vi "1-Tap 8-Bit Camera with Centroid (Host).vi"() -> ()   [LabVIEW 2012]
doc: "This is the host VI for the 1-Tap 8-Bit Camera with Centroid example. This example demonstrates how to perform image processing operations on the FPGA in real time and display the results on the host. This example performs an image thresholding operation followed by a centroid computation. The threshold parameters can be modified using the controls on the front panel. The thresholded images and centroid coordinates are displayed in real time.\n\nAdditionally, the example demonstrates the serial server, which allows third-party camera configuration utilities to communicate with the camera using the Camera Link serial interface while this VI is running."
uses:
  <vilib>/userdefined/High Color/nirio_resource_hc.ctl
  <vilib>/FPGAPlugInAG/PCIe-1473R/niLvFpga_Open_PCIe-1473R.vi
  <vilib>/rvi/interface/common/dynamic/niFpgaDynamicAddResources.vi
  <vilib>/FPGAPlugInAG/Dynamic/niLvFpga_Reset_Dynamic.vi
  <vilib>/Utility/error.llb/Error Cluster From Error Code.vi
  <vilib>/rvi/errors/niLvFpgaAdjustHostInterfaceError.vi
  <vilib>/FPGAPlugInAG/Dynamic/niLvFpga_Run_Dynamic.vi
  <vilib>/FPGAPlugInAG/Dynamic/niLvFpga_Close_Dynamic.vi
  <vilib>/rvi/interface/nirviOpenFPGA/nirviOpenFPGA.xnode
  FPGA Bitfiles/1-Tap8-BitCamera_FPGATarget_1-Tap8-BitCamera_B0CF732A.lvbitx
  1-Tap 8-Bit Camera with Centroid (FPGA).vi
  <vilib>/rvi/interface/nirviMethod/nirviMethod.xnode
  <vilib>/rvi/interface/nirviReadWriteControl/nirviReadWriteControl.xnode
  <vilib>/rvi/interface/nirviCloseFPGA/nirviCloseFPGA.xnode
  NiFpgaLv.dll
  <vilib>/rvi/interface/Simulation/niFpgaSimulationCallBeginRW.vi
  <vilib>/FPGAPlugInAG/Dynamic/niLvFpga_ConfigureFifo_Dynamic.vi
  <vilib>/rvi/errors/niLvFpgaMergeErrorWithErrorCode.vi
  <vilib>/FPGAPlugInAG/Dynamic/niLvFpga_StartFifo_Dynamic.vi
  <vilib>/FPGAPlugInAG/Dynamic/niLvFpga_ReadFifo_Dynamic.vi
panel:
  in  "Invert Image":bool
  out "Y Centroid":fxp<+,32,16> format="%.21g"
  out "X Centroid":fxp<+,32,16> format="%.21g"
  in  "Replace?":bool
  in  "Replace Value":u8=255
  in  "Lower Limit":u8=128
  in  "Upper Limit":u8=255
  out "Acq In Progress":bool
  in  "Line Scan":bool
  in  "Frames To Acquire":u32=1 caption="Frames To Acquire\n(0 = infinite)"
  in  "Cancel":bool
  out "Acq'd Frame Width":u32
  in  "Stopped":bool
  in  "RIO Device":T1="RIO0"
  out "DMA Write Timeout":bool
  in  "Start Serial Server":bool=TRUE
  out "Frames Acq'd":u32
  out "Acq'd Frame Height":u32
  out "Image":T2(plugin-control)
  in  "Acquire":bool
  in  "Stop":bool
  in  "Image Height":u32=480 max=65535
  in  "Image Width":u32=640 max=65535
  out "Initialized":bool
  # "Note: For the centroid, the image must be a light object\non dark background, or you can invert the image."
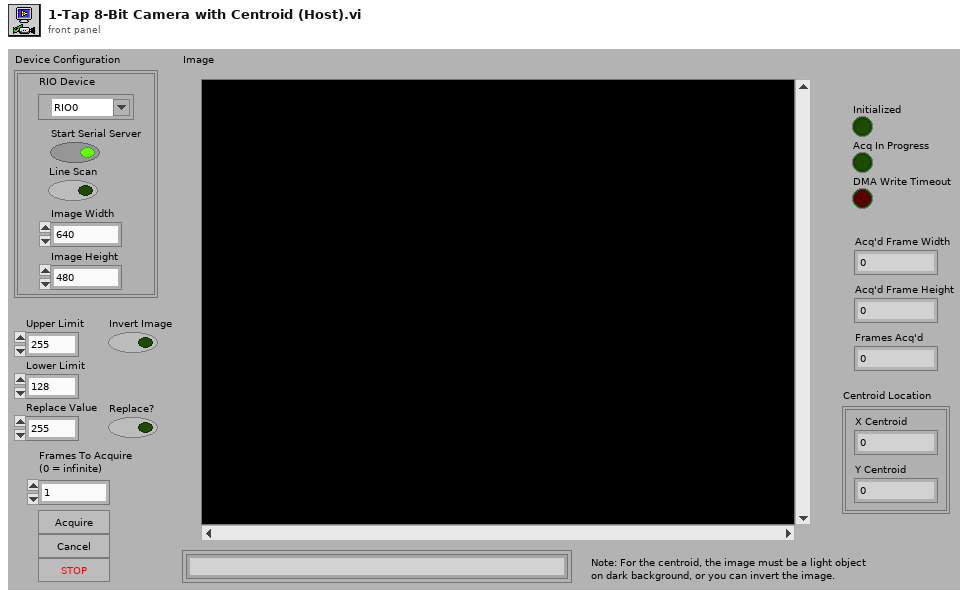
[diagram p1: front panel]
types:
  T1 = typedef "nirio_resource_hc.ctl" = tag
  T2 = typedef "IMAQ Image.ctl" = refnum<image>
  T3 = enum8{"Standard", "Basler 10-tap", "Vosskühler 10-tap"}
  T4 = typedef "Image Type" = u32
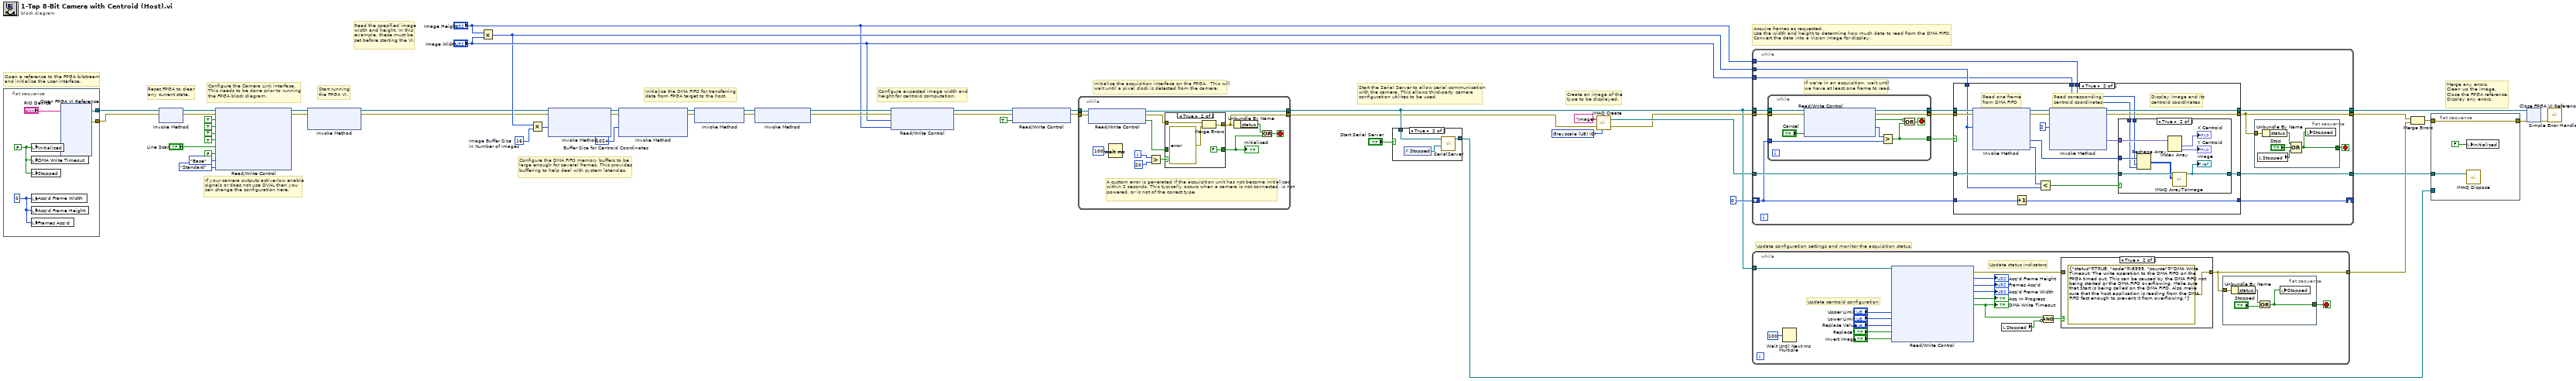
[diagram p0: block diagram]
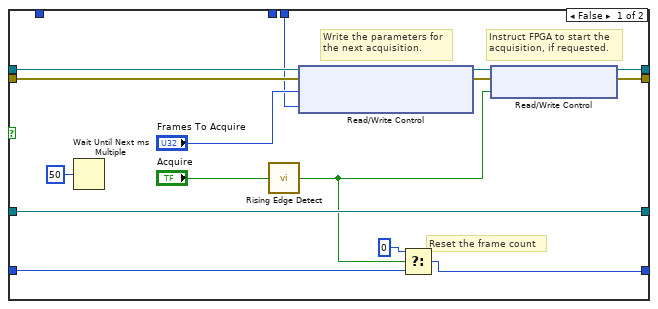
[diagram p4: hidden frame]
diagram:
  w10 = 1024  # Buffer Size for Centroid Coordinates
  w47 = T4 0 items=["Grayscale (U8)", "Grayscale (I16)", "Grayscale (SGL)", "Complex (CSG)", "RGB (U32)", "HSL (U32)", "RGB (U64)", "Grayscale (U16)"] ("Image Type")
  w28 = u32 16  # Image Buffer Size in Number of Images
  # "Configure expected image width and\nheight for centroid computation."
  # "If your camera outputs active-low enable\nsignals or does not use DVAL then you\ncan change the configuration here."
  # "Configure the DMA FIFO memory buffers to be\nlarge enough for several frames. This provides\nbuffering to help deal with system latencies."
  # "Start running\nthe FPGA VI."
  # "Reset FPGA to clear\nany current state."
  # "Read the specified image\nwidth and height. In this\nexample, these must be\nset before starting the VI."
  # "Merge any errors.\nClean up the image.\nClose the FPGA reference.\nDisplay any errors."
  # "Acquire frames as requested.\nUse the width and height to determine how much data to read from the DMA FIFO.\nConvert the data into a Vision Image for display."
  # "Update configuration settings and monitor the acquisition status."
  # "Start the Serial Server to allow serial communication\nwith the camera. This allows third-party camera\nconfiguration utilites to be used."
  # "Create an image of the\ntype to be displayed."
  # "Initialize the acquisition interface on the FPGA.  This will\nwait until a pixel clock is detected from the camera."
  # "Initialize the DMA FIFO for transferring\ndata from FPGA target to the host."
  # "Configure the Camera Link interface.\nThis needs to be done prior to running\nthe FPGA block diagram."
  # "Open a reference to the FPGA bitstream\nand initialize the user interface."
  n1 = flat-sequence {
    tunnel: [w53] -> w43
    tunnel: [w52] -> w51
    frame #0 {
      w56 = u32 0 ("Num Lines Acq'd")
      w55 = FALSE ("stop")
      n2 = local write "Initialized"(w55) -> ()
      n3 = local write "DMA Write Timeout"(w55) -> ()
      n4 = local write "Stopped"(w55) -> ()
      n5 = local write "Acq'd Frame Width"(w56) -> ()
      n6 = local write "Acq'd Frame Height"(w56) -> ()
      n7 = local write "Frames Acq'd"(w56) -> ()
      n8 = xnode "Open FPGA VI Reference"("resource name"="RIO Device") -> ("FPGA VI Reference Out"=w53:refnum<k20>, "error out"=w52:errorcluster)  [unwired: 1 in]
    }
  }
  n9 = xnode "Invoke Method"("FPGA VI Reference In"=w43, "error in"=w51) -> ("FPGA VI Reference Out"=w35:refnum<k20>, "error out"=w38:errorcluster)
  n10 = xnode "Read/Write Control"("FPGA VI Reference In"=w35, "error in"=w38, "CL Config.FVAL Active High"=TRUE ("IO Module Config.CL FVAL Active High"), "CL Config.LVAL Active High"=TRUE ("IO Module Config.CL LVAL Active High"), "CL Config.DVAL Active High"=TRUE ("IO Module Config.CL DVAL Active High"), "CL Config.Spare Active High"=TRUE ("IO Module Config.CL Spare Active High"), "CL Config.Line Scan"="Line Scan", "Acq Control.Ignore DVAL"=FALSE ("CL Config.Line Scan"), "CL Config.Configuration"=enum8{"Base", "Medium", "Full"}."Base", "CL Config.Signal Mapping"=T3."Standard") -> ("FPGA VI Reference Out"=w39:refnum<k20>, "error out"=w37:errorcluster)
  n11 = xnode "Invoke Method"("FPGA VI Reference In"=w39, "error in"=w37) -> ("FPGA VI Reference Out"=w2:refnum<k20>, "error out"=w1:errorcluster)  [unwired: 1 in]
  n12 = Multiply(x="Image Height", y="Image Width") -> (x*y=w11:u32)
  n13 = Multiply(x=w11, y=w28) -> (x*y=w30:u32)
  n14 = xnode "Invoke Method"("FPGA VI Reference In"=w2, "error in"=w1, "Requested Depth"=w30) -> ("FPGA VI Reference Out"=w23:refnum<k20>, "error out"=w20:errorcluster)  [unwired: 1 out]
  n15 = xnode "Invoke Method"("FPGA VI Reference In"=w23, "error in"=w20, "Requested Depth"=w10) -> ("FPGA VI Reference Out"=w22:refnum<k20>, "error out"=w19:errorcluster)  [unwired: 1 out]
  n16 = xnode "Invoke Method"("FPGA VI Reference In"=w22, "error in"=w19) -> ("FPGA VI Reference Out"=w21:refnum<k20>, "error out"=w18:errorcluster)
  n17 = xnode "Invoke Method"("FPGA VI Reference In"=w21, "error in"=w18) -> ("FPGA VI Reference Out"=w17:refnum<k20>, "error out"=w16:errorcluster)
  n18 = xnode "Read/Write Control"("FPGA VI Reference In"=w17, "error in"=w16, "Centroid.Image Width"="Image Width", "Centroid.Image Height"="Image Height") -> ("FPGA VI Reference Out"=w13:refnum<k20>, "error out"=w12:errorcluster)
  n19 = xnode "Read/Write Control"("FPGA VI Reference In"=w13, "error in"=w12, "Acq Control.Initialize"=TRUE ("Arm Acquisition")) -> ("FPGA VI Reference Out"=w50:refnum<k20>, "error out"=w49:errorcluster)
  n20 = while {
    tunnel: w50 -> [w64]
    tunnel: w49 -> [w63]
    tunnel: [w62] -> w27
    tunnel: [w66] -> w26
    i -> [w58]
    stop <- w69 stop-if-true
    # "A custom error is generated if the acquisition unit has not become initialized within 2 seconds. This typically occurs when a camera is not connected, is not powered, or is not of the correct type."
    n21 = xnode "Read/Write Control"("FPGA VI Reference In"=w64, "error in"=w63) -> ("FPGA VI Reference Out"=w62:refnum<k20>, "error out"=w61:errorcluster, "Acq Status.Initialized"=w60:bool)
    n22 = Wait (ms)(milliseconds to wait=u32 100) -> ()  [unwired: 1 out]
    n23 = Greater?(x=w58, y=20) -> (0:w59:bool)
    n24 = case shown="True" w59 {
      tunnel: [w71 FALSE] -> w65
      tunnel: w60 -> [w71 _]
      tunnel: w61 -> [w70 w73]
      tunnel: [w70 w75] -> w66
      frame False {
      }
      frame True {
        n25 = Merge Errors(w73, errorcluster {"status"=TRUE, "code"=-8999, "source"="Acquisition Initialization: This error typically occurs when a camera is not properly connected, is not powered, or is not of the correct type."} ("error in")) -> (w75:errorcluster)
      }
    }
    "Initialized" <- w65
    n26 = Unbundle By Name(w66) -> ("status"=w68:bool)
    n27 = Or(x=w68, y=w65) -> (x .or. y?=w69:bool)
  }
  n28 = case shown="True" "Start Serial Server" {
    tunnel: [_ w76] -> w44
    tunnel: w27 -> [_ w77]
    frame False {
    }
    frame True {
      n29 = control-ref of="Stopped"() -> (w78:refnum<vi>)
      n30 = call "SerialServer.vi"("Stop Refnum"=w78, "FPGA VI Reference In"=w77) -> ("FPGA VI Reference Out"=w76:refnum<k20>)  [unwired: 5 in]
    }
  }
  n31 = call "IMAQ Create"("Image Name"="Image", "Image Type"=w47, "error in (no error)"=w26) -> ("New Image"=w6:T2, "error out"=w5:errorcluster)  [unwired: 2 in]
  n32 = while {
    tunnel: w27 -> [w85]
    tunnel: w5 -> [w84]
    tunnel: w11 -> [w93]
    tunnel: "Image Height" -> [w92]
    tunnel: "Image Width" -> [w91]
    tunnel: w6 -> [w90]
    tunnel: [w88] -> w41
    tunnel: [w89] -> w9
    tunnel: [w86] -> w45
    shift-right: [w80] -> _
    shift-left: u32 0 -> [w79]
    stop <- w87 stop-if-true
    # "If we're in an acquisition, wait until\nwe have at least one frame to read."
    n33 = while {
      tunnel: w85 -> [w100]
      tunnel: w84 -> [w99]
      tunnel: [w97] -> w83
      tunnel: [w98] -> w82
      tunnel: w79 -> [w103]
      tunnel: [w101] -> w81
      stop <- w102 stop-if-true
      n34 = xnode "Read/Write Control"("FPGA VI Reference In"=w100, "error in"=w99, "Acq Control.Cancel Acq"="Cancel") -> ("FPGA VI Reference Out"=w98:refnum<k20>, "error out"=w97:errorcluster, "Acq Status.Acq In Progress"=w96:bool, "Acq Status.Frames Acq'd"=w95:u32)
      n35 = Greater?(x=w95, y=w103) -> (0:w101:bool)
      n36 = Compound Arithmetic op=OR(invert w96, w101) -> (w102:bool)
    }
    n37 = case shown="True" w81 {
      tunnel: w82 -> [w119 w139]
      tunnel: w83 -> [w118 w138]
      tunnel: w93 -> [_ w127]
      tunnel: w92 -> [w116 w125]
      tunnel: w91 -> [_ w124]
      tunnel: w90 -> [w123 w141]
      tunnel: [w112 w131] -> w88
      tunnel: [w115 w132] -> w89
      tunnel: [w123 w140] -> w86
      tunnel: w79 -> [w120 w137]
      tunnel: [w122 w136] -> w80
      frame False {
        # "Reset the frame count"
        # "Instruct FPGA to start the\nacquisition, if requested."
        # "Write the parameters for\nthe next acquisition."
        n38 = Wait Until Next ms Multiple(millisecond multiple=u32 50) -> ()  [unwired: 1 out]
        n39 = call "Rising Edge Detect.vi"("Input"="Acquire") -> ("Pulse"=w109:bool)  [unwired: 4 in]
        n40 = xnode "Read/Write Control"("FPGA VI Reference In"=w119, "error in"=w118, "Acq Control.Frames To Acq"="Frames To Acquire", "Acq Control.Line Scan Height"=w116) -> ("FPGA VI Reference Out"=w114:refnum<k20>, "error out"=w113:errorcluster)
        n41 = Select(t=u32 0, s=w109, f=w120) -> (s? t:f=w122:u32)
        n42 = xnode "Read/Write Control"("FPGA VI Reference In"=w114, "error in"=w113, "Acq Control.Acquire"=w109) -> ("FPGA VI Reference Out"=w115:refnum<k20>, "error out"=w112:errorcluster)
      }
      frame True {
        # "Read corresponding\ncentroid coordinates"
        # "Display image and its\ncentroid coordinates"
        # "Read one frame\nfrom DMA FIFO"
        n43 = xnode "Invoke Method"("FPGA VI Reference In"=w139, "error in"=w138, "Number of Elements"=w127) -> ("FPGA VI Reference Out"=w134:refnum<k20>, "error out"=w133:errorcluster, "Data"=w135:u8[], "Elements Remaining"=w128:u32)  [unwired: 1 in]
        n44 = Increment(x=w137) -> (x+1=w136:u32)
        n45 = Less?(x=w128, y=w127) -> (x < y?=w126:bool)
        n46 = xnode "Invoke Method"("FPGA VI Reference In"=w134, "error in"=w133, "Number of Elements"=u32 2) -> ("FPGA VI Reference Out"=w132:refnum<k20>, "error out"=w131:errorcluster, "Data"=w129:fxp<+,32,16>[])  [unwired: 1 in, 1 out]
        n47 = case shown="True" w126 {
          tunnel: w141 -> [w142 w151]
          tunnel: [w142 w150] -> w140
          tunnel: w135 -> [_ w149]
          tunnel: w129 -> [_ w147]
          tunnel: w125 -> [_ w144]
          tunnel: w124 -> [_ w143]
          frame False {
            # "Do not display the image if we're\nfalling behind in the acquisition."
          }
          frame True {
            n48 = Reshape Array(w149, w144, w143) -> (w148:u8[][])
            n49 = Index Array(array=w147) -> (element #1=→"X Centroid":fxp<+,32,16>, element #2=→"Y Centroid":fxp<+,32,16>)  [unwired: 2 in]
            n50 = call "IMAQ ArrayToImage"("Image Pixels (U8)"=w148, "Image"=w151) -> ("Image Out"=w150:T2)  [unwired: 8 in, 1 out]
            "Image" <- w150
          }
        }
      }
    }
    n51 = flat-sequence {
      tunnel: w88 -> [w106]
      tunnel: [w105] -> w87
      frame #0 {
        n52 = local read "Stopped"() -> (w104:bool)
        n53 = Unbundle By Name(w106) -> ("status"=w107:bool)
        n54 = Compound Arithmetic op=OR(w107, "Stop", w104) -> (w105:bool)
        n55 = local write "Stopped"(w105) -> ()
      }
    }
  }
  n56 = while {
    tunnel: w27 -> [w165]
    tunnel: [w168] -> w40
    stop <- w167 stop-if-true
    # "Update centroid configuration"
    # "Update status indicators"
    n57 = Wait Until Next ms Multiple(millisecond multiple=u32 100) -> ()  [unwired: 1 out]
    n58 = xnode "Read/Write Control"("FPGA VI Reference In"=w165, "Threshold.Upper Limit"="Upper Limit", "Threshold.Lower Limit"="Lower Limit", "Threshold.Replacement"="Replace Value", "Threshold.Replace"="Replace?", "Threshold.Invert"="Invert Image") -> ("error out"=w164:errorcluster, "Acq Status.Lines Per Frame"=→"Acq'd Frame Height":u32, "Acq Status.Frames Acq'd"=→"Frames Acq'd":u32, "Acq Status.Clocks Per Line"=→"Acq'd Frame Width":u32, "Acq Status.Acq In Progress"=→"Acq In Progress":bool, "Acq Status.DMA Write Timeout"=w153:bool)  [unwired: 1 in, 1 out]
    "DMA Write Timeout" <- w153
    n59 = local read "Stopped"() -> (w154:bool)
    n60 = Compound Arithmetic op=AND(w153, invert w154) -> (w152:bool)
    n61 = case shown="True" w152 {
      tunnel: w164 -> [w173 _]
      tunnel: [w173 errorcluster {"status"=TRUE, "code"=-8999, "source"="DMA Write Timeout: The write operation to the DMA FIFO on the FPGA timed out. This can be caused by the DMA FIFO not being started or the DMA FIFO overflowing. Make sure that Start is being called on the DMA FIFO. Also make sure that the host application is reading from the DMA FIFO fast enough to prevent it from overflowing."} ("error out")] -> w168
      frame False {
      }
      frame True {
      }
    }
    n62 = flat-sequence {
      tunnel: w168 -> [w172]
      tunnel: [w170] -> w167
      frame #0 {
        n63 = Unbundle By Name(w172) -> ("status"=w171:bool)
        n64 = Or(x=w171, y="Stopped") -> (x .or. y?=w170:bool)
        n65 = local write "Stopped"(w170) -> ()
      }
    }
  }
  n66 = Merge Errors(w41, w40) -> (w42:errorcluster)
  n67 = flat-sequence {
    tunnel: w42 -> [w176]
    tunnel: [w176] -> w7
    tunnel: w45 -> [w177]
    tunnel: w44 -> [_]
    frame #0 {
      n68 = local write "Initialized"(FALSE ("Module Enabled")) -> ()
      n69 = call "IMAQ Dispose"("Image"=w177) -> ()  [unwired: 5 in, 1 out]
    }
  }
  n70 = xnode "Close FPGA VI Reference"("FPGA VI Reference In"=w9, "error in"=w7) -> ("error out"=w8:errorcluster)
  n71 = call <vilib>:"Simple Error Handler.vi"("error in (no error)"=w8) -> ()  [unwired: 4 in, 5 out]
